vi "Main - Fan Characterisation - Steady State - [Student].vi"() -> ()   [LabVIEW 2017]
uses:
  <vilib>/Utility/file.llb/Read Delimited Spreadsheet (DBL).vi
  <vilib>/Analysis/NI_AALPro.lvlib
  <vilib>/ptbypt/NI_PtbyPt.lvlib
panel:
  out "Averaging Filter Buffer Length (s)":dbl
  out "Filtered Thrust Measurement (N)":dbl format="%.4f"
  in  "Zero Offset":bool
  out "Calibration Data - Slope (V/N)":dbl format="%#_3g"
  out "Calibration Data - Intersect (V)":dbl format="%#_4g"
  out "Force Measurement":cluster{"mean":dbl, dbl}(graph)
  in  "Fan Control Signal":dbl min=0.0 max=10.0 step=0.5
  out "Load Cell Calibration Data":cluster{"Y":dbl[], "Y":dbl[]}[](graph)
  in  "stop":bool
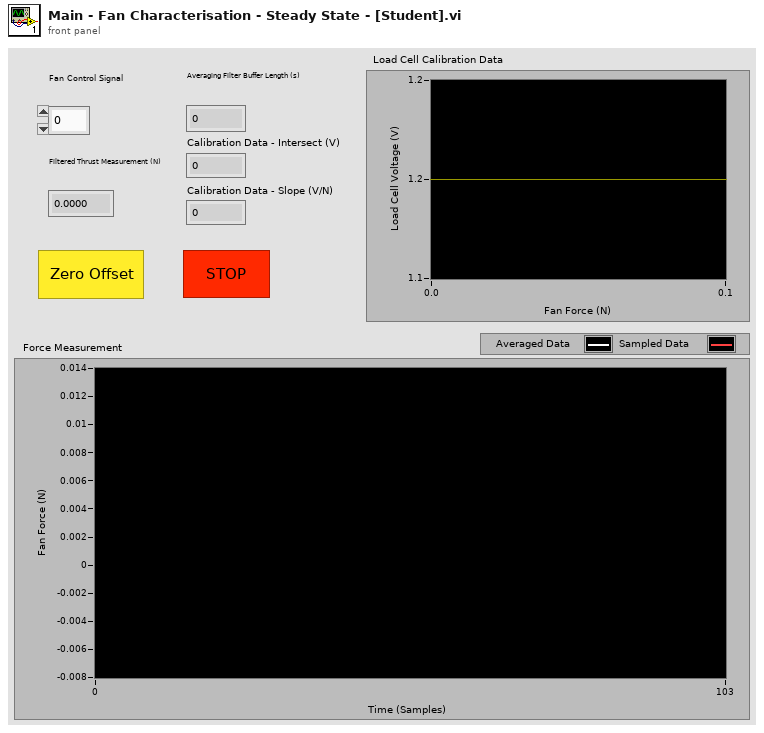
[diagram p1: front panel]
types:
  T1 = cluster{"AI Task":refnum<k21>, "Ctr0 Task":refnum<k21>, "Ao Task":refnum<k21>, "DO Task":refnum<k21>}
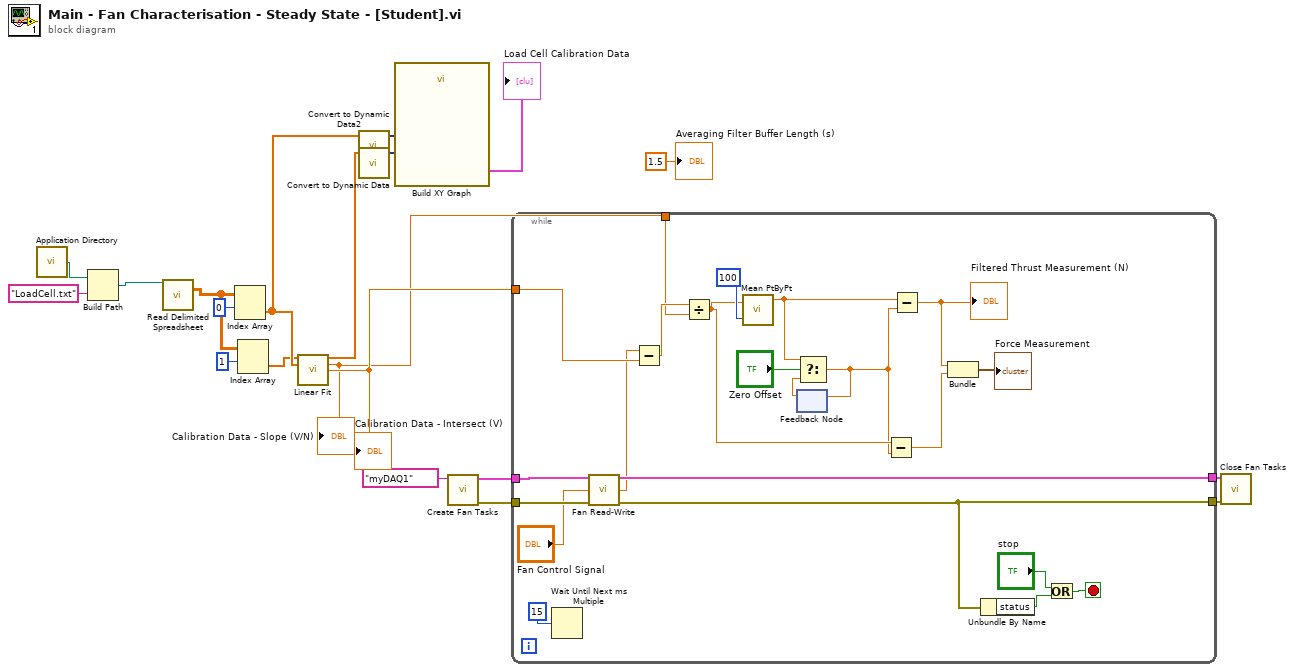
[diagram p0: block diagram]
diagram:
  n1 = call <vilib>:"Application Directory.vi"() -> ("Application Directory"=w9:path)
  n2 = Build Path(base path=w9, name or relative path="LoadCell.txt") -> (appended path=w8:path)
  n3 = call-poly <vilib>:"Read Delimited Spreadsheet.vi"("file path (dialog if empty)"=w8) -> ("all rows"=w11:dbl[][])  [unwired: 9 in, 5 out]
  n4 = Index Array(array=w11, index (row)=0) -> (element=w14:dbl[])  [unwired: 1 in]
  n5 = Index Array(array=w11, index (row)=1) -> (element=w12:dbl[])  [unwired: 1 in]
  n6 = call <vilib>:"Linear Fit.vi"("Y"=w12, "X"=w14) -> ("Best Linear Fit"=w1:dbl[], "slope"=w3:dbl, "intercept"=w4:dbl)  [unwired: 9 in, 2 out]
  "Calibration Data - Intersect (V)" <- w4
  "Calibration Data - Slope (V/N)" <- w3
  n7 = call "Convert to Dynamic Data2"("Array"=w14) -> ("Dynamic Data Type"=w15:dynamicdata)  [unwired: 3 in]
  n8 = call "Convert to Dynamic Data"("Array"=w1) -> ("Dynamic Data Type"=w13:dynamicdata)  [unwired: 3 in]
  n9 = call "Build XY Graph"("Y Input"=w13, "X Input"=w15) -> ("XY Graph"=→"Load Cell Calibration Data":cluster{"X":dbl[], "Y":dbl[]}[])  [unwired: 8 in, 1 out]
  n10 = call "Create Fan Tasks.vi"("DAQmx Device Name"=tag "myDAQ1") -> ("Error Out"=w19:errorcluster, "Hellicopter Tasks Output"=w20:T1)  [unwired: 5 in]
  n11 = while {
    tunnel: w20 -> [w41]
    tunnel: w19 -> [w42]
    tunnel: [w40] -> w18
    tunnel: [w37] -> w17
    tunnel: w4 -> [w33]
    tunnel: w3 -> [w30]
    stop <- w39 stop-if-true
    n12 = Wait Until Next ms Multiple(millisecond multiple=u32 15) -> ()  [unwired: 1 out]
    n13 = call "Fan Read-Write.vi"("Hellicopter Tasks Input"=w41, "Fan Input"="Fan Control Signal", "Error In"=w42) -> ("Hellicopter Tasks Output"=w40:T1, "L/C Output"=w32:dbl, "Error Out"=w37:errorcluster)  [unwired: 10 in]
    n14 = Subtract(x=w32, y=w33) -> (x-y=w31:dbl)
    n15 = Divide(x=w31, y=w30) -> (x/y=w24:dbl)
    n16 = call <vilib>:"Mean PtByPt.vi"("x"=w24, "sample length"=100) -> ("mean"=w22:dbl)  [unwired: 2 in, 1 out]
    n17 = feedback #1() -> (w28:dbl)  [unwired: 1 in]
    n18 = Select(t=w22, s="Zero Offset", f=w28) -> (s? t:f=w23:dbl)
    n19 = feedback-in #1(w23) -> ()
    n20 = Subtract(x=w24, y=w23) -> (x-y=w25:dbl)
    n21 = Subtract(x=w22, y=w23) -> (x-y=w21:dbl)
    "Filtered Thrust Measurement (N)" <- w21
    n22 = Bundle(w21, w25) -> (→"Force Measurement":cluster{dbl, dbl})  [unwired: 1 in]
    n23 = Unbundle By Name(w37) -> ("status"=w36:bool)
    n24 = Or(x="stop", y=w36) -> (x .or. y?=w39:bool)
  }
  n25 = call "Close Fan Tasks.vi"("Error In"=w17, "Hellicopter Tasks Input 2"=w18) -> ()  [unwired: 9 in, 1 out]
  "Averaging Filter Buffer Length (s)" <- 1.5 ("Averaging Filter Buffer Length (s)")
